vi "Pneumatic Press and Hold.vi"   [LabVIEW 2013]
uses:
  State Machine Enum.ctl
  <vilib>/Rock Robotics/WPI/Solenoid/WPI_SolenoidValue.ctl
  <vilib>/Rock Robotics/WPI/Solenoid/WPI_SolenoidSetEnum.vi
  Robot Global Data.vi
types:
  T1 = typedef "State Machine Enum.ctl" = enum16{"Init", "Actuate", "Retract"}
  T2 = typedef "WPI_SolenoidValue.ctl" = enum16{"Off", "On", "Forward", "Reverse"}
  T3 = typedef "WPI_SolenoidDevRef.ctl" = cluster{"DevStatus":errorcluster, "Solenoid Module":T4, "Forward Solenoid Channel":T5, "Reverse Solenoid Channel":T5}
  T4 = typedef "FPGA_TypedefSolenoidModule.ctl" = enum16{"Solenoid Module 1", "Solenoid Module 2"}
  T5 = typedef "WPI_SolenoidChannel.ctl" = enum8{"Solenoid 1", "Solenoid 2", "Solenoid 3", "Solenoid 4", "Solenoid 5", "Solenoid 6", "Solenoid 7", "Solenoid 8", "Invalid"}
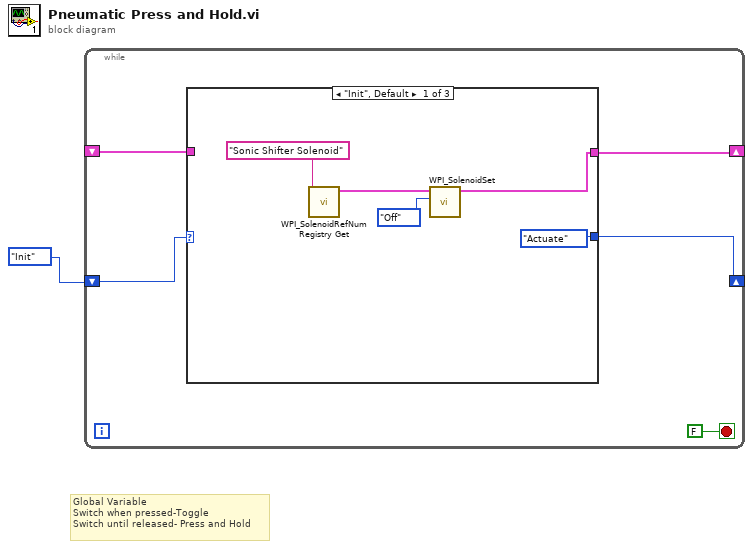
[diagram p0: block diagram]
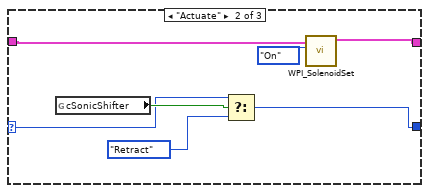
[diagram p2: hidden frame]
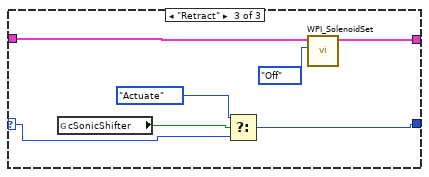
[diagram p3: hidden frame]
diagram:
  # "Global Variable\nSwitch when pressed-Toggle\nSwitch until released- Press and Hold"
  n1 = while {
    shift-right: [w5] -> _
    shift-left: State_Machine_Enum."Init" -> [w6]
    shift-right: [w4] -> _
    shift-left: _ -> [w3]
    stop <- FALSE stop-if-true
    n2 = case shown="\"Init\", Default" w6 {
      selector: w6 -> [_ w12 w19]
      tunnel: [State_Machine_Enum."Actuate" w14 w20] -> w5
      tunnel: [w8 w18 w22] -> w4
      tunnel: w3 -> [_ w17 w23]
      frame "Init", Default {
        n3 = call <vilib>:"WPI_SolenoidRefNum Registry Get.vi"("refnum name"="Sonic Shifter Solenoid") -> ("SolenoidDevRef"=w9:T3)  [unwired: 9 in, 1 out]
        n4 = call-poly <vilib>:"WPI_SolenoidSet.vi"("Value"=WPI_SolenoidValue."Off", "SolenoidDevRef"=w9) -> ("SolenoidDevRef"=w8:T3)  [unwired: 8 in, 1 out]
      }
      frame "Actuate" {
        n5 = global read "Robot Global Data.vi" "cSonicShifter"() -> (w16:bool)
        n6 = Select(t=w12, s=w16, f=State_Machine_Enum."Retract") -> (s? t:f=w14:T1)
        n7 = call-poly <vilib>:"WPI_SolenoidSet.vi"("Value"=WPI_SolenoidValue."On", "SolenoidDevRef"=w17) -> ("SolenoidDevRef"=w18:T3)  [unwired: 8 in, 1 out]
      }
      frame "Retract" {
        n8 = global read "Robot Global Data.vi" "cSonicShifter"() -> (w25:bool)
        n9 = Select(t=State_Machine_Enum."Actuate", s=w25, f=w19) -> (s? t:f=w20:T1)
        n10 = call-poly <vilib>:"WPI_SolenoidSet.vi"("Value"=WPI_SolenoidValue."Off", "SolenoidDevRef"=w23) -> ("SolenoidDevRef"=w22:T3)  [unwired: 8 in, 1 out]
      }
    }
  }
